vi "GUI_HTT_MultiCamDriveGaiaProfile.vi"() -> ()   [LabVIEW 2020]
uses:
  Shared/GUI_Template/GUI_master/tcp_new_data_event.ctl
  Shared/GUI_Template/GUI_master/tcp new data cluster.ctl
  General GUIs/Device GUIs/GUI_Cameras/Controls/Crosshair type def.ctl
  <userlib>/_OpenG.lib/array/array.llb/Filter 1D Array with Scalar (String)__ogtk.vi
panel:
  out "String 4":string="x1\ny1\nx2\ny2"
  out "String 3":string="x1\ny1\nx2\ny2"
  out "String 2":string="x1\ny1\nx2\ny2"
  out "String":string="x1\ny1\nx2\ny2"
  in  "visibility":bool=TRUE
  out "appended array":string[](array[string]) caption="XH"
  out "appended array 6":string[](array[string]) caption="XH"
  out "appended array 8":string[](array[string]) caption="XH"
  out "appended array 4":string[](array[string]) caption="XH"
  in  "UDP error message":string
  out "tcp data event 2":T1
  out "error IO 2":errorcluster
  in  "Color Box":u32(colorbox)
  in  "TargetSize.Y::3":dbl=163.0 caption="y" min=2.0 max=3000.0 format="%#_6f"
  in  "TargetSize.X::3":dbl=152.0 caption="x" min=2.0 max=3000.0 format="%#_6f"
  in  "TargetSize.Y::2":dbl=74.0 caption="y" min=2.0 max=3000.0 format="%#_6f"
  in  "TargetSize.X::2":dbl=75.0 caption="x" min=2.0 max=3000.0 format="%#_6f"
  in  "active cams":string
  out "CCDs":string[](array[string])
  out "Cameras":T2
  in  "Target.Y::3":dbl=163.0 caption="y" min=0.0 max=2000.0 format="%#_6f"
  in  "Target.X::3":dbl=152.0 caption="x" min=0.0 max=2000.0 format="%#_6f"
  in  "Target.Y::2":dbl=74.0 caption="y" min=0.0 max=2000.0 format="%#_6f"
  in  "Target.X::2":dbl=75.0 caption="x" min=0.0 max=2000.0 format="%#_6f"
  out "error out":errorcluster
  in  "triggerdelay::3":dbl=0.001 caption="triggerdelay" min=0.0 max=10000000.0 format="%_4p"
  in  "triggerdelay::2":dbl=0.001 caption="triggerdelay" min=0.0 max=10000.0 format="%_4p"
  in  "centroidy::5":dbl=0.001 caption="centroid y" min=0.0 max=0.0 format="%_4f"
  in  "centroidx::5":dbl=0.001 caption="centroid x" min=0.0 max=0.0 format="%_4f"
  in  "trigger::3":bool caption="Trigger"
  in  "centroidy::3":dbl=0.001 caption="centroid y" min=0.0 max=0.0 format="%_4f"
  in  "centroidx::3":dbl=0.001 caption="centroid x" min=0.0 max=0.0 format="%_4f"
  in  "exposure::3":dbl=0.001 caption="exposure" min=1e-07 max=5.0 format="%_4p"
  out "image::3":T3(plugin-control) caption="HTT-MagCam-03"
  in  "GUIdevice 3":string="HTT-C24_1_gmode_n"
  in  "trigger::2":bool caption="Trigger"
  in  "centroidy::2":dbl=0.001 caption="centroid y" min=0.0 max=0.0 format="%_4f"
  in  "centroidx::2":dbl=0.001 caption="centroid x" min=0.0 max=0.0 format="%_4f"
  in  "exposure::2":dbl=0.001 caption="exposure" min=0.0001 max=1.0 format="%_4p"
  out "image::2":T3(plugin-control) caption="HTT-MagCam-04"
  in  "GUIdevice 2":string="HTT-C13_4_gmode_s"
  out "tcp data event":T1
  in  "Refresh Button":bool caption="Update Crosshairs"
  in  "Select device":string(combo)="FrogHPD"
  in  "stop":bool
  in  "GUIdevice 1":string="HPD_CCD"
  # "XHair location"
  # "XHair location"
  # "XHair size"
  # "XHair size"
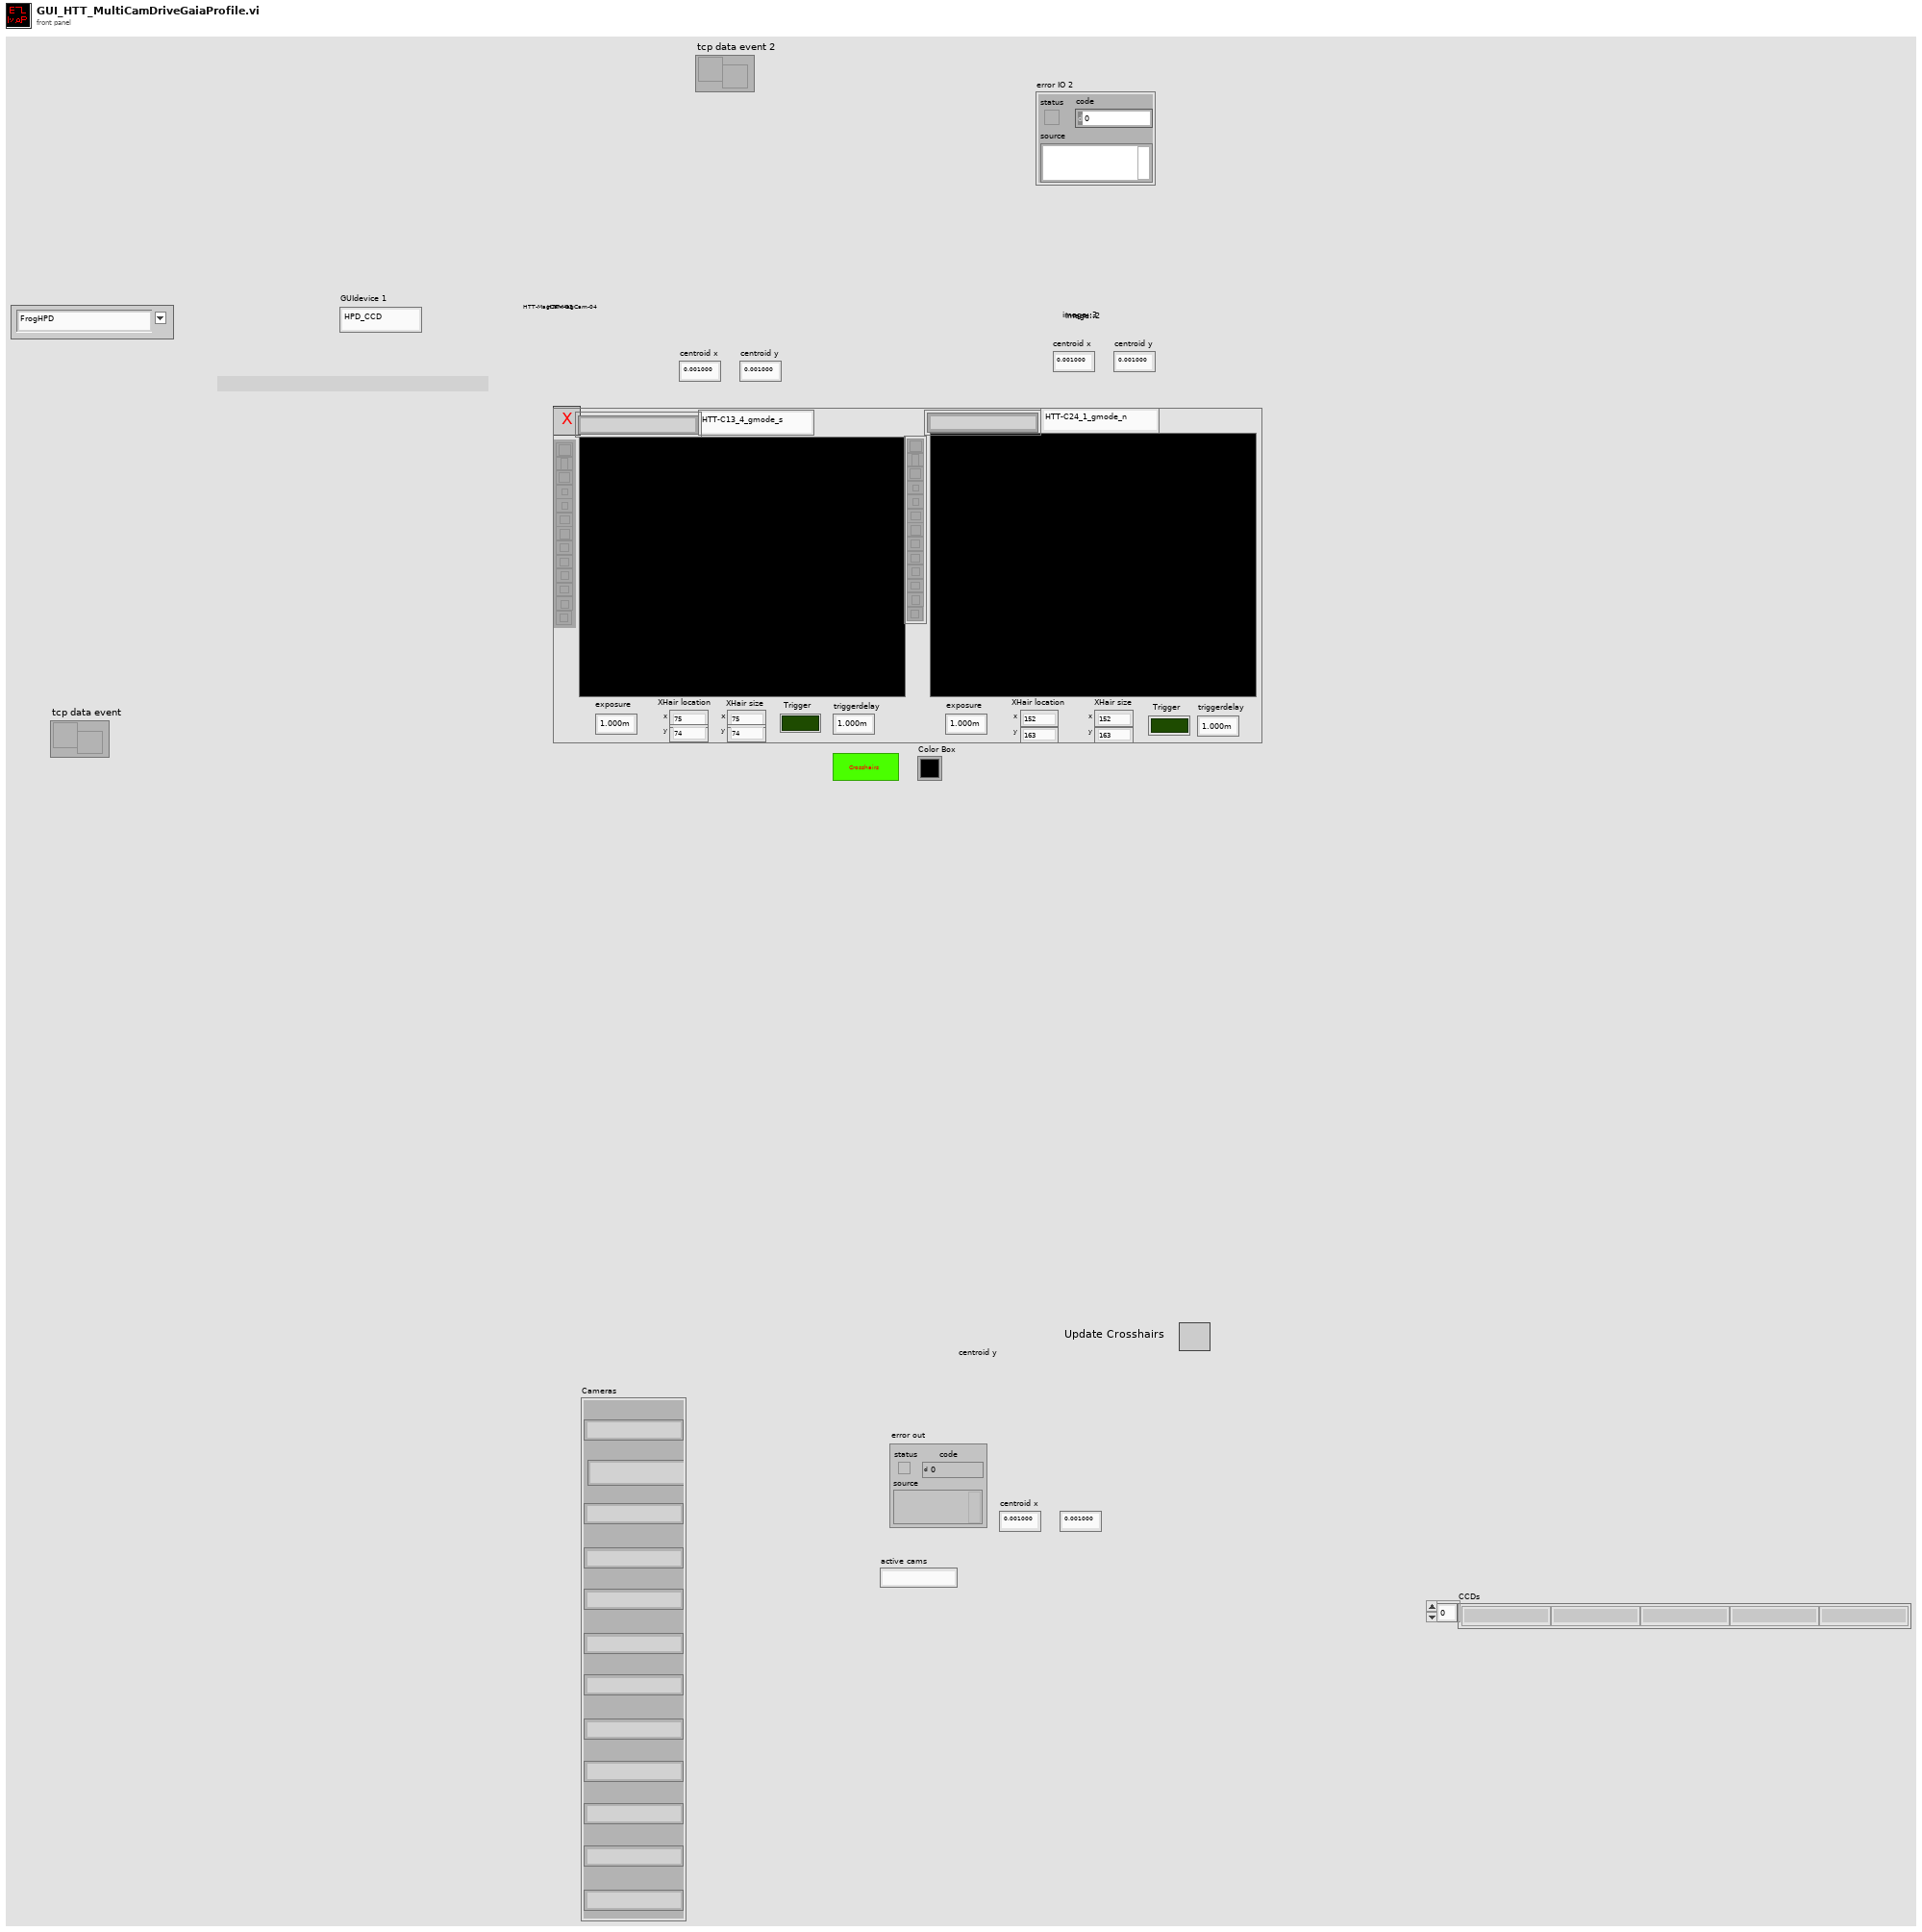
[diagram p1: front panel]
types:
  T1 = typedef "tcp_new_data_event.ctl" = refnum<user-event>
  T2 = cluster{"[0]":string, "[1]":string, "[2]":string, "[3]":string, "[4]":string, "[5]":string, "[6]":string, "[7]":string, "[8]":string, "[8] 2":string, "[8] 3":string, "[8] 4":string}
  T3 = typedef "IMAQ Image.ctl" = refnum<image>
  T4 = typedef "Image Type" = u32
  T5 = cluster{"Target.X::2":refnum<vi>, "Target.Y::2":refnum<vi>}
  T6 = cluster{"Target.X::3":refnum<vi>, "Target.Y::3":refnum<vi>}
  T7 = cluster{"TargetSize.X::2":refnum<vi>, "TargetSize.Y::2":refnum<vi>}
  T8 = cluster{"TargetSize.X::3":refnum<vi>, "TargetSize.Y::3":refnum<vi>}
  T9 = cluster{"Target.X::3":refnum<vi>, "Target.Y::3":refnum<vi>}[]
  T10 = cluster{"TargetSize.X::3":refnum<vi>, "TargetSize.Y::3":refnum<vi>}[]
  T11 = cluster{"[0]":string, "[1]":string, "[2]":string, "[3]":string, "[4]":string, "[5]":string, "[6]":string, "[7]":string, "[8]":string, "[9]":string, "[10]":string, "[11]":string}
  T12 = typedef "Crosshair type def.ctl" = cluster{"Draw":bool, "Target":cluster{"x":dbl, "y":dbl}, "Size":cluster{"x":dbl, "y":dbl}, "Angle":dbl, "Color":u32, "Thickness":u8, "CrosshairLabel":string}
  T13 = cluster{"Left":i32, "Top":i32, "Right":i32, "Bottom":i32}
  T14 = enum32{"invalid app kind", "Development System", "Run Time System", "Student Edition", "Embedded LabVIEW", "Evaluation", "Custom"}
  T15 = typedef "tcp new data cluster.ctl" = cluster{"EventEnum":enum16{"new data", "connection status update"}, "Device name":string}
  T16 = enum32{"Invalid", "Standard", "Closed", "Hidden", "Minimized", "Maximized"}
  T17 = cluster{"Core":cluster{"Current VI Reference":refnum<vi>, "Close Panel on Exit?":bool}, "Your Boolean data":bool, "active cams":string, "SuperGUI":cluster{"STOP queue":refnum<queue>, "SuperGUI ref":refnum<vi>}}
  T18 = cluster{"STOP queue":refnum<queue>, "SuperGUI ref":refnum<vi>}
  T19 = cluster{"Current VI Reference":refnum<vi>, "Close Panel on Exit?":bool}
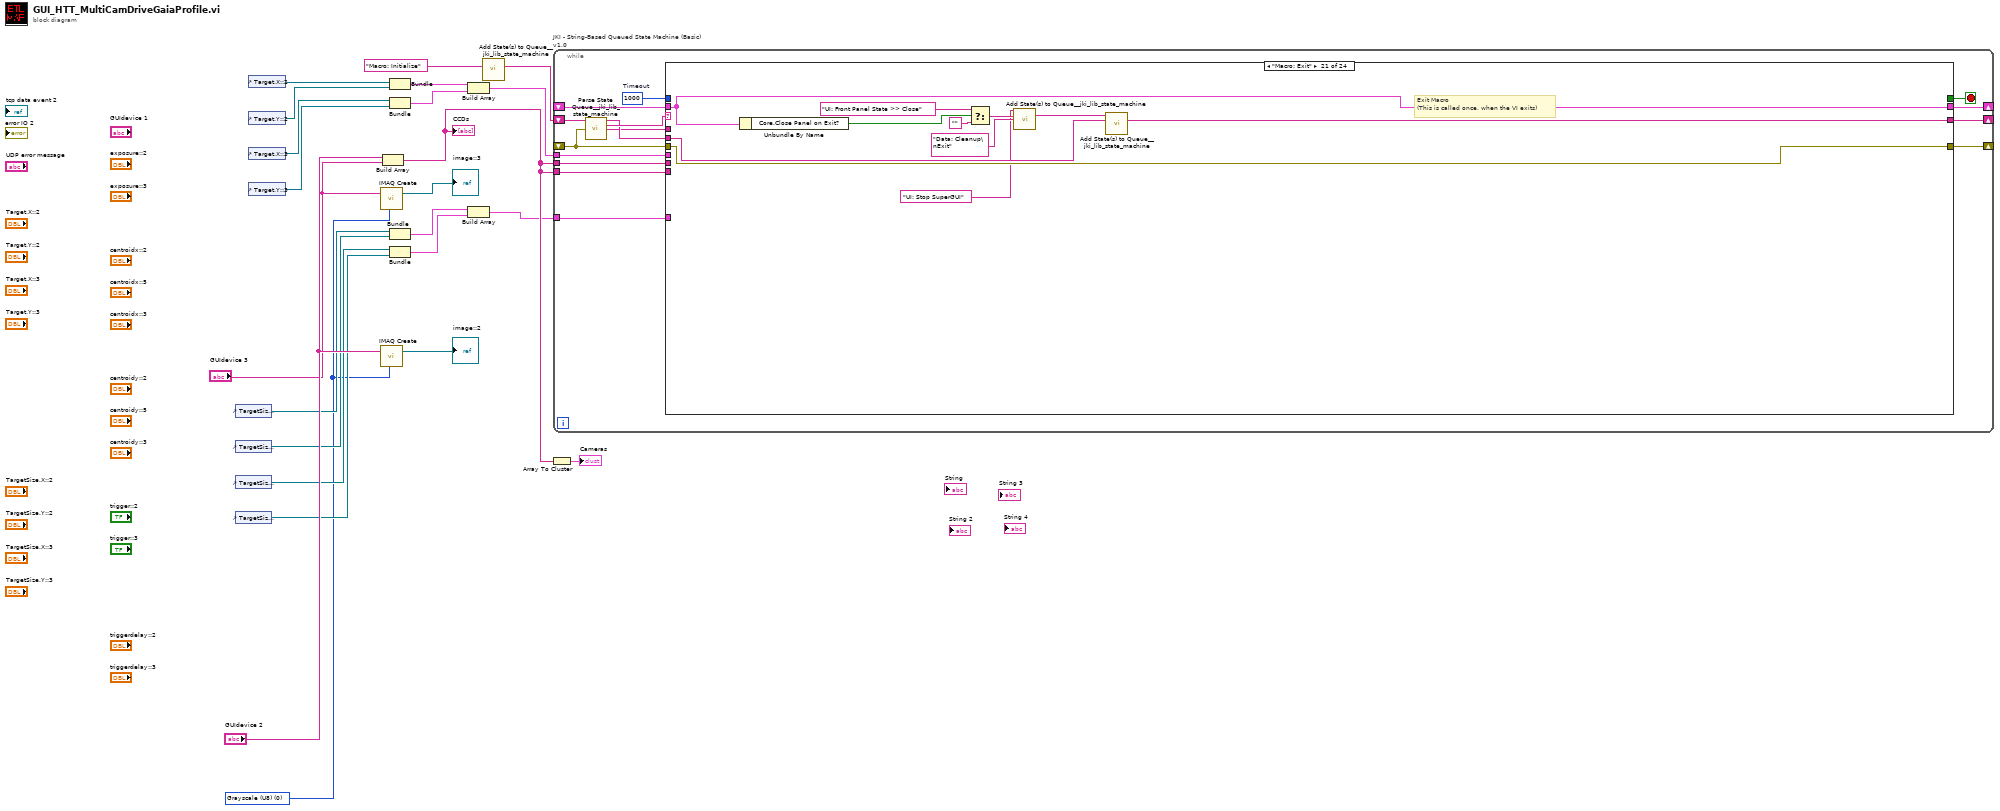
[diagram p0: block diagram]
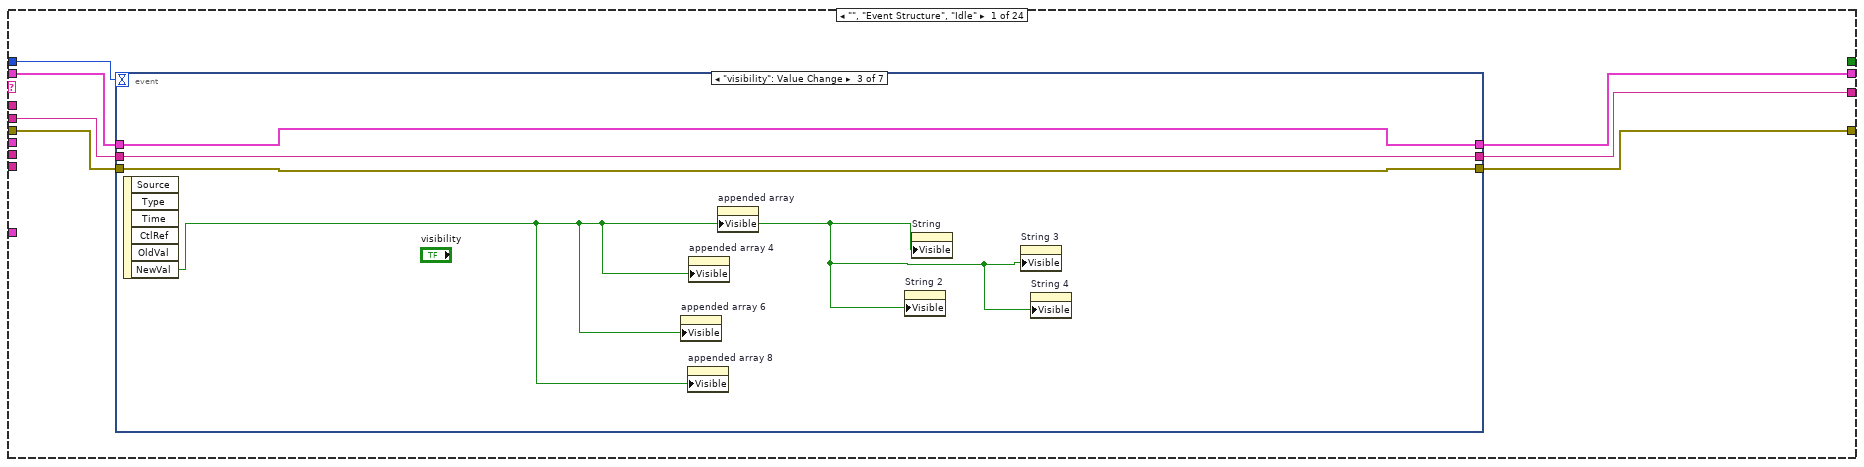
[diagram p2: hidden frame]
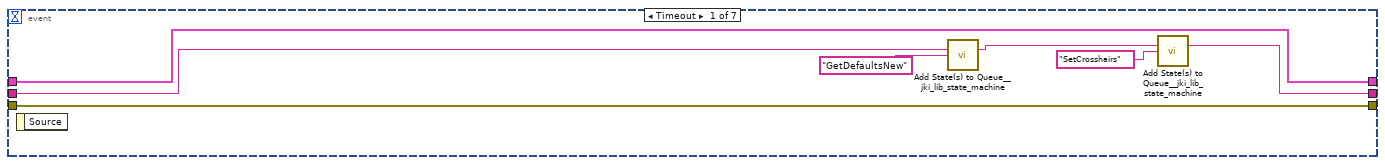
[diagram p3: hidden frame]
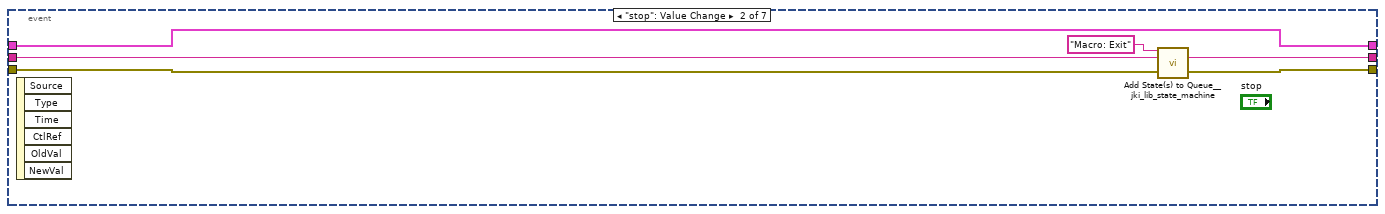
[diagram p4: hidden frame]
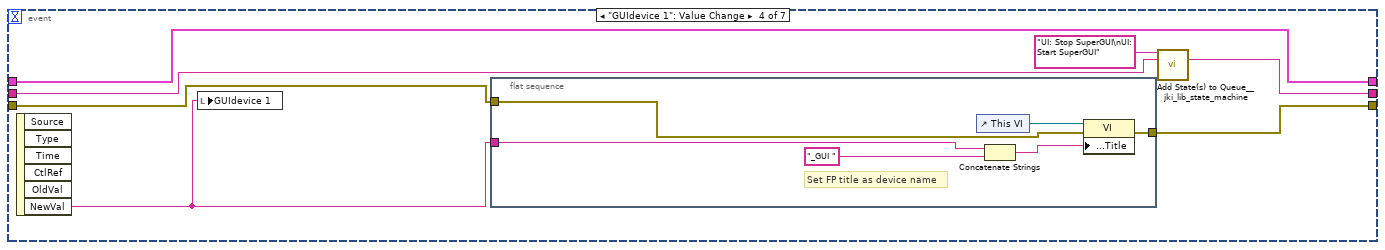
[diagram p5: hidden frame]
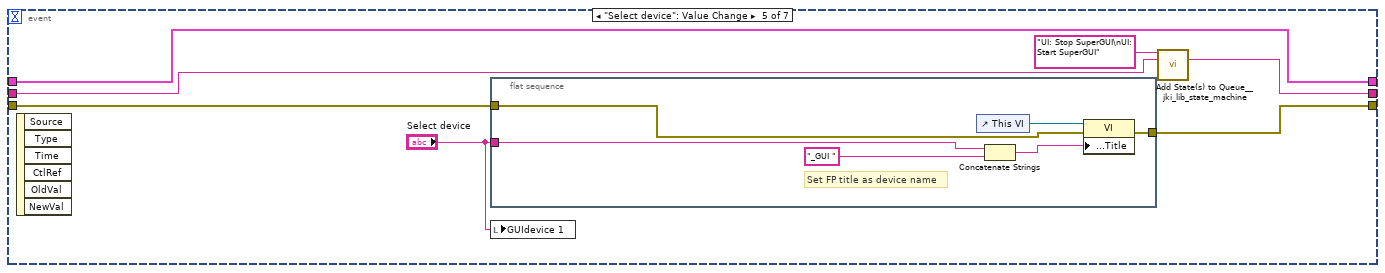
[diagram p6: hidden frame]
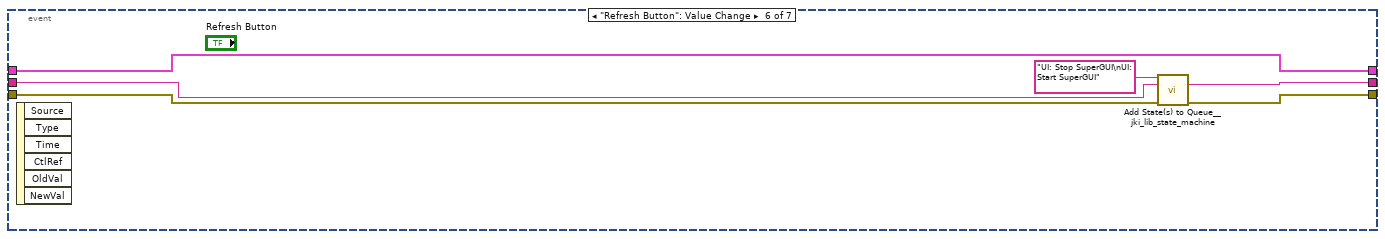
[diagram p7: hidden frame]
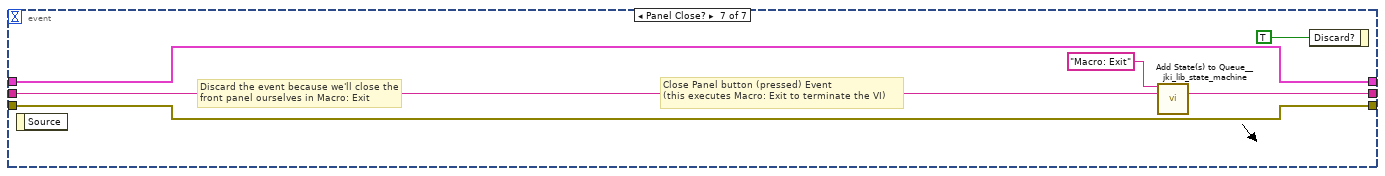
[diagram p8: hidden frame]
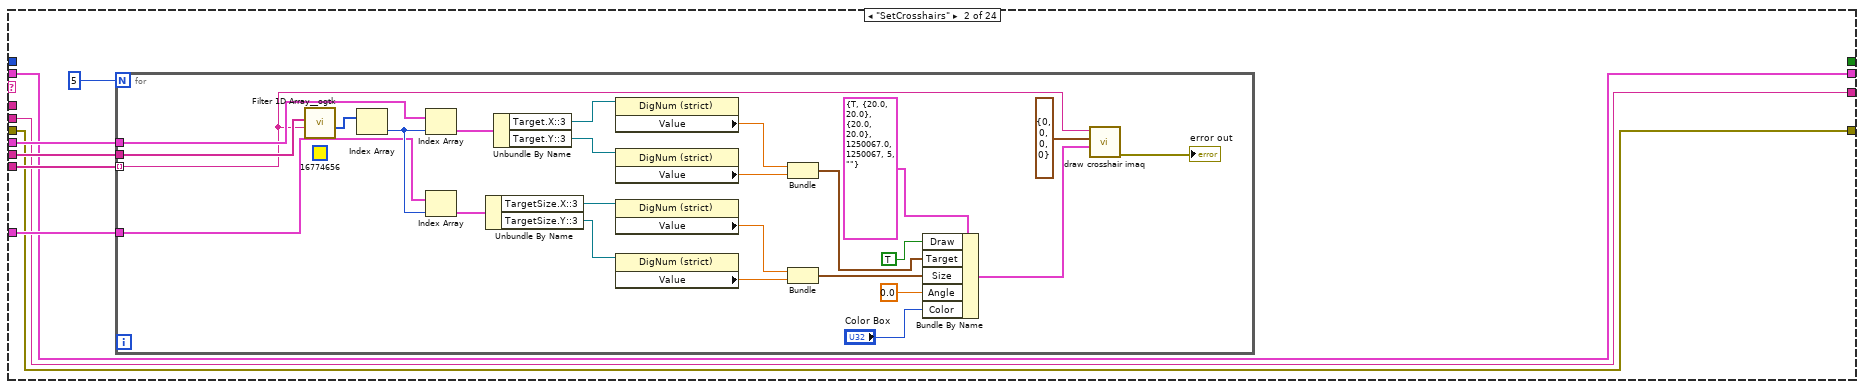
[diagram p9: hidden frame]
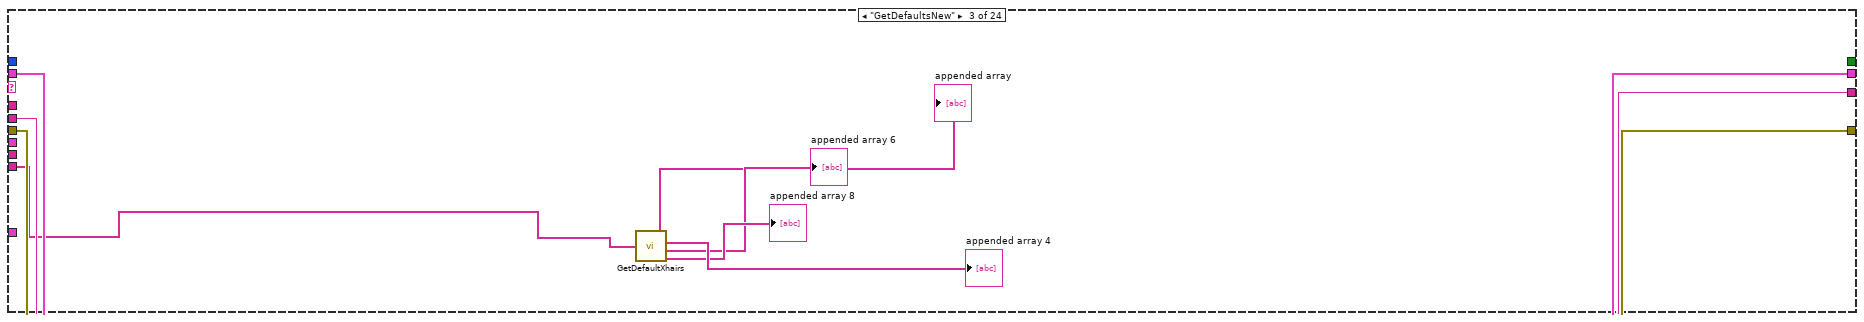
[diagram p10: hidden frame]
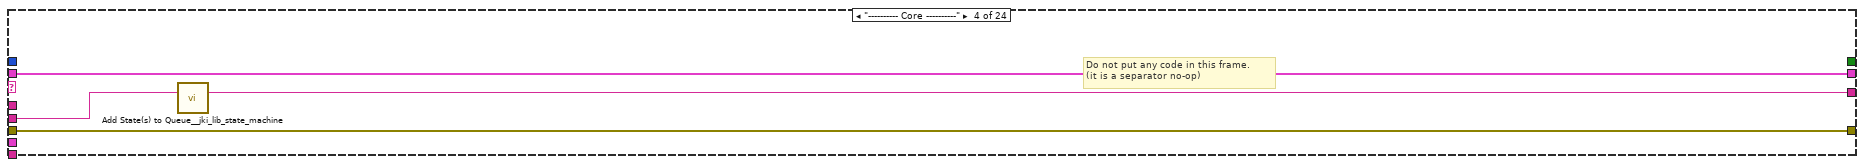
[diagram p11: hidden frame]
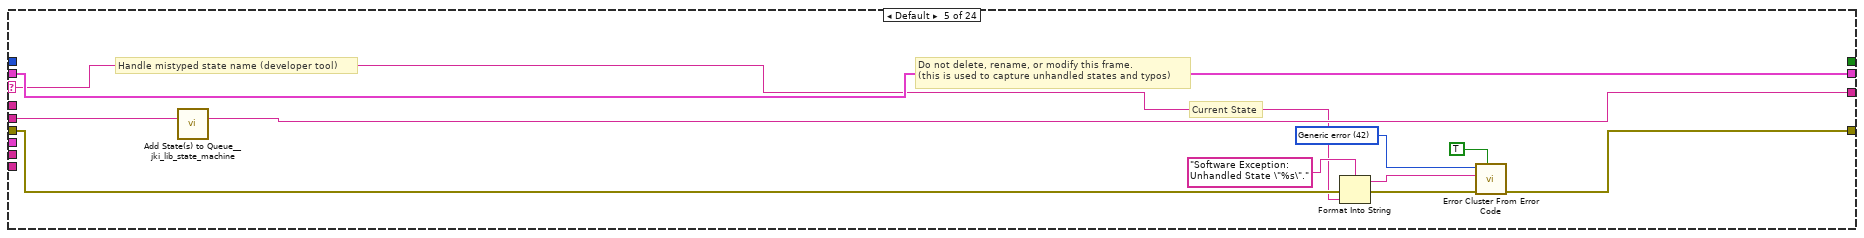
[diagram p12: hidden frame]
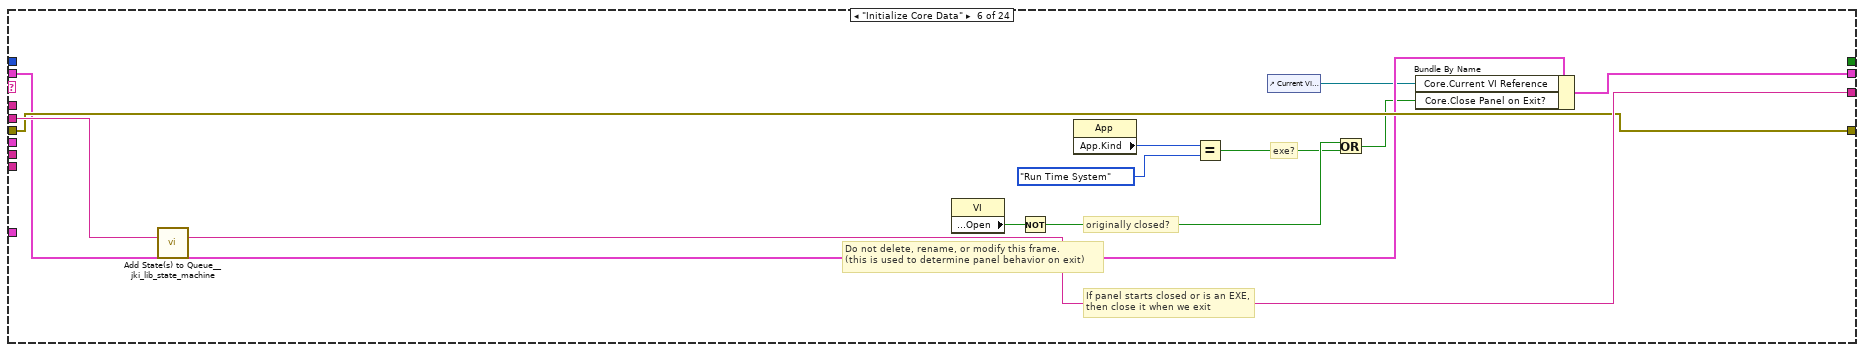
[diagram p13: hidden frame]
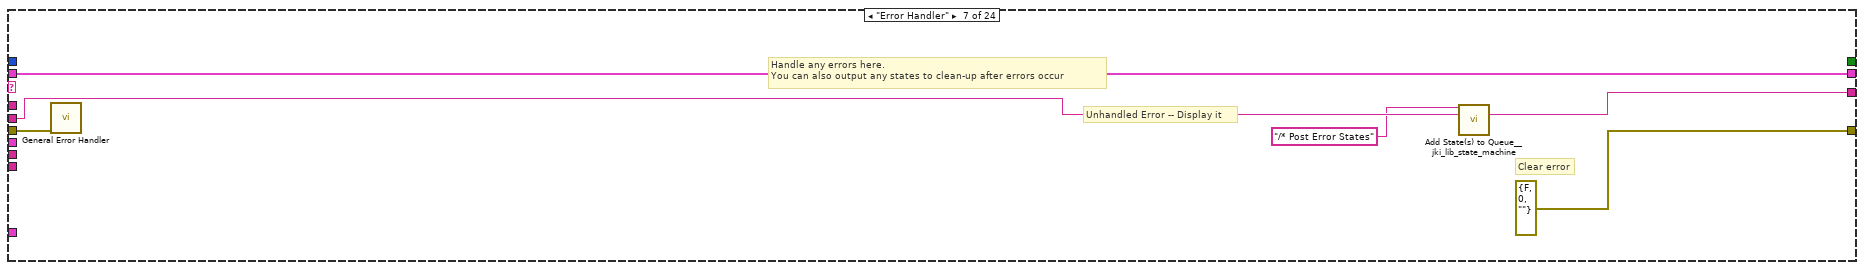
[diagram p14: hidden frame]
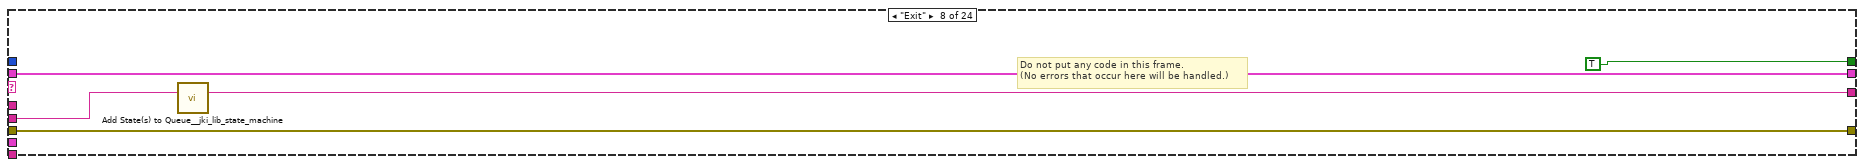
[diagram p15: hidden frame]
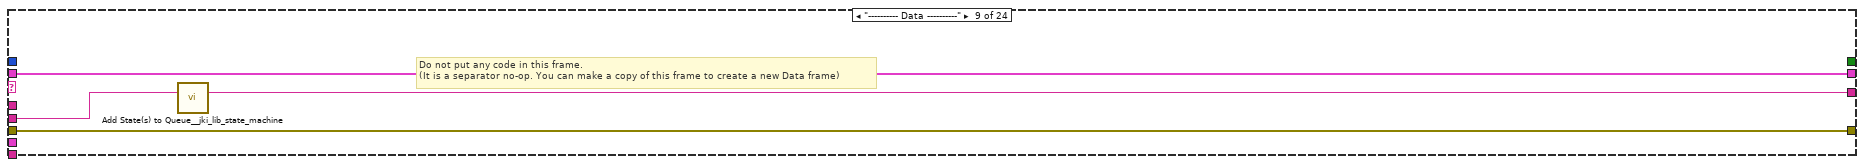
[diagram p16: hidden frame]
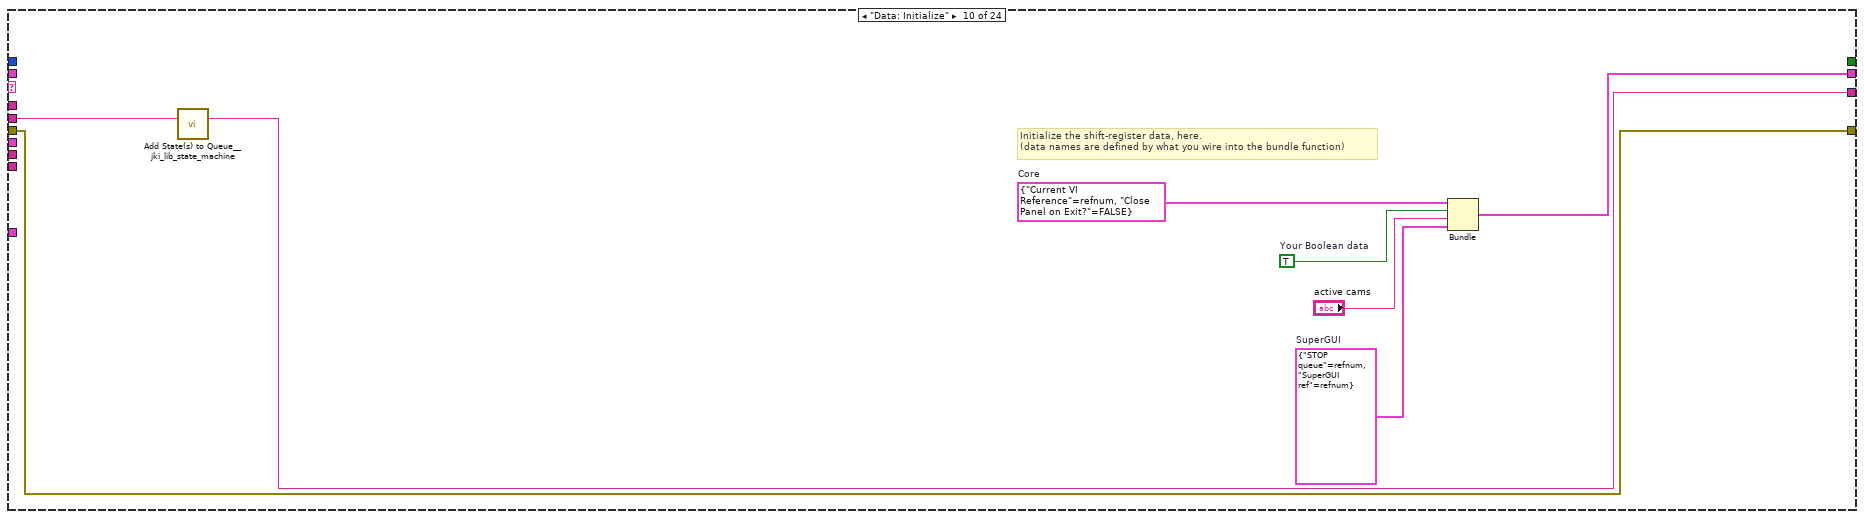
[diagram p17: hidden frame]
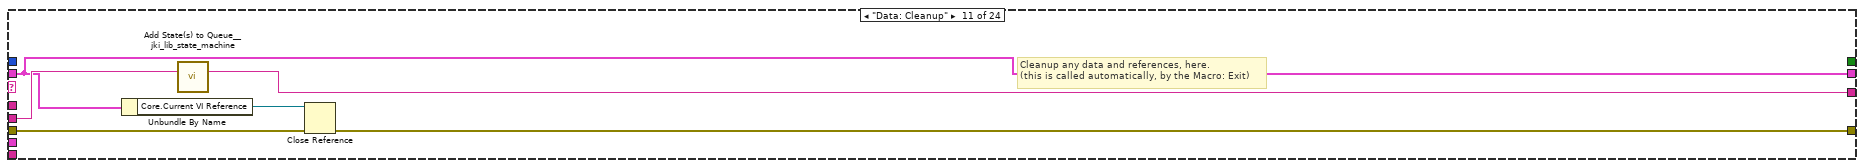
[diagram p18: hidden frame]
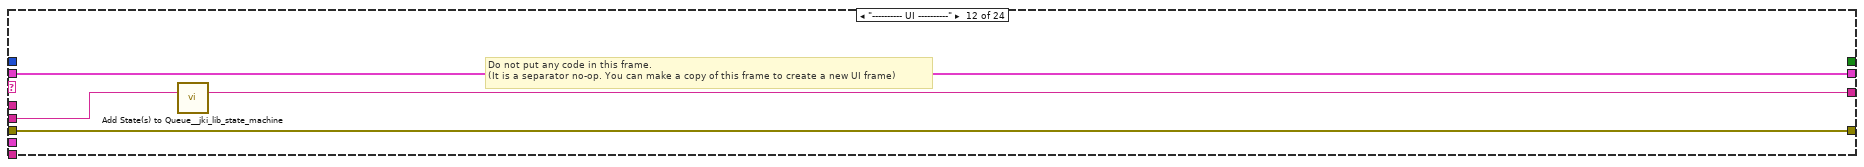
[diagram p19: hidden frame]
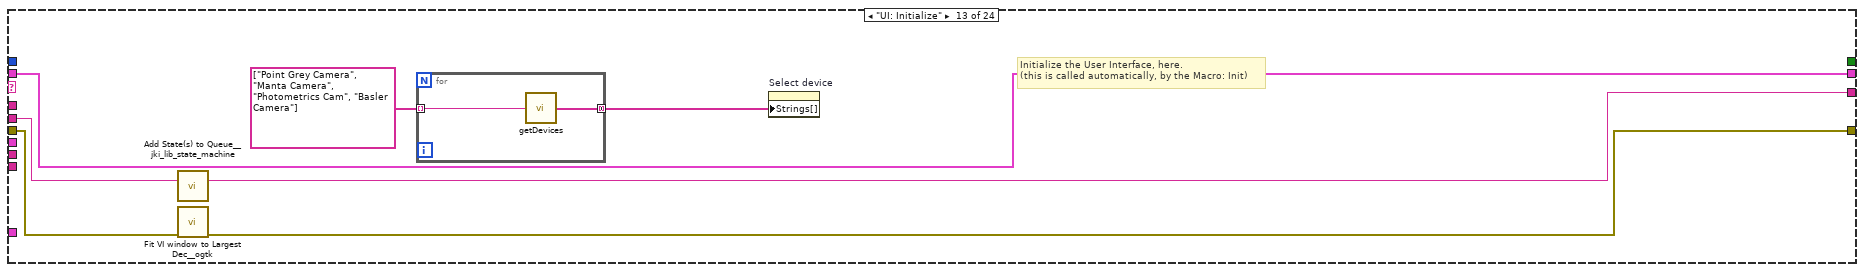
[diagram p20: hidden frame]
diagram:
  w1 = T4 0 items=["Grayscale (U8)", "Grayscale (I16)", "Grayscale (SGL)", "Complex (CSG)", "RGB (U32)", "HSL (U32)", "RGB (U64)", "Grayscale (U16)"] ("Image Type")
  n1 = control-ref of="TargetSize.X::2"() -> (w8:refnum<vi>)
  n2 = control-ref of="TargetSize.Y::2"() -> (w7:refnum<vi>)
  n3 = control-ref of="TargetSize.X::3"() -> (w6:refnum<vi>)
  n4 = control-ref of="TargetSize.Y::3"() -> (w5:refnum<vi>)
  n5 = control-ref of="Target.X::2"() -> (w19:refnum<vi>)
  n6 = control-ref of="Target.Y::2"() -> (w18:refnum<vi>)
  n7 = control-ref of="Target.X::3"() -> (w17:refnum<vi>)
  n8 = control-ref of="Target.Y::3"() -> (w16:refnum<vi>)
  n9 = call "IMAQ Create"("Image Name"="GUIdevice 3", "Image Type"=w1) -> ("New Image"=→"image::3":T3)  [unwired: 3 in, 1 out]
  n10 = call "IMAQ Create"("Image Name"="GUIdevice 2", "Image Type"=w1) -> ("New Image"=→"image::2":T3)  [unwired: 3 in, 1 out]
  n11 = Build Array("GUIdevice 2", "GUIdevice 3") -> (w9:string[])
  "CCDs" <- w9
  n12 = Bundle("Target.X::2"=w19, "Target.Y::2"=w18) -> (w15:T5)  [unwired: 1 in]
  n13 = Bundle("Target.X::3"=w17, "Target.Y::3"=w16) -> (w14:T6)  [unwired: 1 in]
  n14 = Bundle("TargetSize.X::2"=w8, "TargetSize.Y::2"=w7) -> (w4:T7)  [unwired: 1 in]
  n15 = Bundle("TargetSize.X::3"=w6, "TargetSize.Y::3"=w5) -> (w3:T8)  [unwired: 1 in]
  n16 = Build Array(w15, w14) -> (w13:T9)
  n17 = Build Array(w4, w3) -> (w2:T10)
  n18 = call <vilib>:"Add State(s) to Queue__jki_lib_state_machine.vi"("State(s) in (\"\")"="Macro: Initialize") -> ("States Out"=w23:string)  [unwired: 14 in]
  n19 = Array To Cluster(array=w9) -> (cluster=→"Cameras":T11)
  n20 = while "JKI - String-Based Queued State Machine (Basic) v1.0" {
    shift-right: [w31] -> _
    shift-left: _ -> [w28]
    shift-right: [w34] -> _
    shift-left: _ -> [w29]
    shift-right: [w33] -> _
    shift-left: w23 -> [w35]
    tunnel: w13 -> [w25]
    tunnel: w9 -> [w26]
    tunnel: w9 -> [w27]
    tunnel: w2 -> [w24]
    stop <- w32 stop-if-true
    w30 = 1000  # Timeout
    n21 = call <vilib>:"Parse State Queue__jki_lib_state_machine.vi"("State Queue"=w35, "Error In (no error)"=w29) -> ("Remaining States"=w37:string, "Current State"=w38:string, "Arguments"=w36:string)  [unwired: 11 in]
    n22 = case shown="\"Macro: Exit\"" w38 {
      selector: w38 -> [_ _ _ _ w144 _ _ _ _ _ _ _ _ _ _ _ _ _ _ _ _ _ _ _]
      tunnel: w37 -> [w45 w101 w138 w143 w148 w166 w172 w177 w181 w189 w195 w199 w206 w214 w249 w257 w263 w274 w300 w305 w316 w320 w324 w328]
      tunnel: w36 -> [_ _ _ _ _ _ _ _ _ _ _ _ _ _ _ _ w258 w268 _ _ _ _ _ _]
      tunnel: w28 -> [w43 w102 w139 w140 w146 w157 w169 w175 w178 _ w190 w196 w204 w212 w240 w252 w261 w270 w297 w302 w313 w317 w321 w325]
      tunnel: [w42 w100 w137 w141 w150 w163 errorcluster {"status"=FALSE, "code"=0, "source"=""} ("error out") w174 w179 w186 w191 w197 w202 w209 w233 w250 w259 w271 w298 w303 w314 w318 w322 w326] -> w34
      tunnel: w29 -> [w41 w100 w137 w141 w149 w163 w168 w174 w179 w186 w192 w197 w203 w210 w234 w251 w260 w272 w298 w303 w314 w318 w322 w326]
      tunnel: [w44 w101 w138 w142 w147 w165 w171 w176 w180 w188 w194 w198 w205 w213 w248 w256 w262 w273 w299 w304 w315 w319 w323 w327] -> w33
      tunnel: [_ _ _ _ _ _ _ TRUE _ _ _ _ _ _ _ _ _ _ _ _ _ _ _ _] -> w32
      tunnel: [w40 w102 w139 w140 w146 w164 w169 w175 w178 w187 w190 w196 w204 w212 w239 w252 w261 w270 w297 w302 w313 w317 w321 w325] -> w31
      tunnel: w30 -> [w39 _ _ _ _ _ _ _ _ _ _ _ _ _ _ _ _ _ _ _ _ _ _ _]
      tunnel: w27 -> [_ w104 w136 _ _ _ _ _ _ _ _ _ _ _ _ _ _ _ _ _ _ _ _ _]
      tunnel: w26 -> [_ w105 _ _ _ _ _ _ _ _ _ _ _ _ _ _ _ _ _ _ _ _ _ _]
      tunnel: w25 -> [_ w106 _ _ _ _ _ _ _ _ _ _ _ _ _ _ _ _ _ _ _ _ _ _]
      tunnel: w24 -> [_ w103 _ _ _ _ _ _ _ _ _ _ _ _ _ _ _ _ _ _ _ _ _ _]
      frame "", "Event Structure", "Idle" {
        n23 = event shown="[2] \"visibility\": Value Change" {
          selector: _ -> [_ _ _ _ _ _ _]
          dyn-events: _ -> [_ _ _ _ _ _ _]
          timeout: w39 -> [_ _ _ _ _ _ _]
          tunnel: w45 -> [w48 w55 w59 w65 w77 w90 w98]
          tunnel: [w52 w54 w59 w64 w76 w89 w97] -> w44
          tunnel: w43 -> [w50 w57 w61 w68 w81 w92 w95]
          tunnel: [w51 w56 w60 w66 w79 w91 w96] -> w42
          tunnel: w41 -> [w51 w56 w60 w67 w80 w91 w96]
          tunnel: [w50 w57 w61 w68 w81 w92 w95] -> w40
          event Timeout {
            n24 = event-data() -> ()  [unwired: 1 in, 1 out]
            n25 = call <vilib>:"Add State(s) to Queue__jki_lib_state_machine.vi"("State(s) in (\"\")"=w48, "State(s) at Back (\"\")"="GetDefaultsNew") -> ("States Out"=w46:string)  [unwired: 13 in]
            n26 = call <vilib>:"Add State(s) to Queue__jki_lib_state_machine.vi"("State(s) in (\"\")"=w46, "State(s) at Back (\"\")"="SetCrosshairs") -> ("States Out"=w52:string)  [unwired: 13 in]
          }
          event "stop": Value Change {
            n27 = event-data() -> ()  [unwired: 1 in, 6 out]
            n28 = call <vilib>:"Add State(s) to Queue__jki_lib_state_machine.vi"("State(s) in Front (\"\")"="Macro: Exit", "State(s) in (\"\")"=w55) -> ("States Out"=w54:string)  [unwired: 13 in]
          }
          event "visibility": Value Change {
            n29 = event-data() -> ("NewVal"=w58:bool)  [unwired: 1 in, 5 out]
            n30 = property on="appended array 6" class="Arr (strict)"("Visible"=w58) -> ()  [unwired: 2 in, 2 out]
            n31 = property on="appended array 8" class="Arr (strict)"("Visible"=w58) -> ()  [unwired: 2 in, 2 out]
            n32 = property on="appended array 4" class="Arr (strict)"("Visible"=w58) -> ()  [unwired: 2 in, 2 out]
            n33 = property on="appended array" class="Arr (strict)"("Visible"=w58) -> ()  [unwired: 2 in, 2 out]
            n34 = property on="String 2" class="Str"("Visible"=w58) -> ()  [unwired: 2 in, 2 out]
            n35 = property on="String" class="Str"("Visible"=w58) -> ()  [unwired: 2 in, 2 out]
            n36 = property on="String 3" class="Str"("Visible"=w58) -> ()  [unwired: 2 in, 2 out]
            n37 = property on="String 4" class="Str"("Visible"=w58) -> ()  [unwired: 2 in, 2 out]
          }
          event "GUIdevice 1": Value Change {
            n38 = event-data() -> ("NewVal"=w62:string)  [unwired: 1 in, 5 out]
            n39 = local write "GUIdevice 1"(w62) -> ()
            n40 = flat-sequence {
              tunnel: [w71] -> w66
              tunnel: w67 -> [w70]
              tunnel: w62 -> [w69]
              frame #0 {
                # "Set FP title as device name"
                n41 = control-ref of="This VI"() -> (w74:refnum<vi>)
                n42 = Concatenate Strings(w69, "_GUI ") -> (w73:string)
                n43 = property class="VI"(reference=w74, error in=w70, "Front Panel.Title"=w73) -> (error out=w71:errorcluster)  [unwired: 1 out]
              }
            }
            n44 = call <vilib>:"Add State(s) to Queue__jki_lib_state_machine.vi"("State(s) in Front (\"\")"="UI: Stop SuperGUI\nUI: Start SuperGUI", "State(s) in (\"\")"=w65) -> ("States Out"=w64:string)  [unwired: 13 in]
          }
          event "Select device": Value Change {
            n45 = event-data() -> ()  [unwired: 1 in, 6 out]
            n46 = flat-sequence {
              tunnel: [w84] -> w79
              tunnel: w80 -> [w83]
              tunnel: "Select device" -> [w82]
              frame #0 {
                # "Set FP title as device name"
                n47 = control-ref of="This VI"() -> (w87:refnum<vi>)
                n48 = Concatenate Strings(w82, "_GUI ") -> (w86:string)
                n49 = property class="VI"(reference=w87, error in=w83, "Front Panel.Title"=w86) -> (error out=w84:errorcluster)  [unwired: 1 out]
              }
            }
            n50 = local write "GUIdevice 1"("Select device") -> ()
            n51 = call <vilib>:"Add State(s) to Queue__jki_lib_state_machine.vi"("State(s) in Front (\"\")"="UI: Stop SuperGUI\nUI: Start SuperGUI", "State(s) in (\"\")"=w77) -> ("States Out"=w76:string)  [unwired: 13 in]
          }
          event "Refresh Button": Value Change {
            n52 = event-data() -> ()  [unwired: 1 in, 6 out]
            n53 = call <vilib>:"Add State(s) to Queue__jki_lib_state_machine.vi"("State(s) in Front (\"\")"="UI: Stop SuperGUI\nUI: Start SuperGUI", "State(s) in (\"\")"=w90) -> ("States Out"=w89:string)  [unwired: 13 in]
          }
          event Panel Close? {
            # "Discard the event because we'll close the front panel ourselves in Macro: Exit"
            # "Close Panel button (pressed) Event\n(this executes Macro: Exit to terminate the VI)"
            n54 = event-data() -> ()  [unwired: 1 in, 1 out]
            n55 = call <vilib>:"Add State(s) to Queue__jki_lib_state_machine.vi"("State(s) in Front (\"\")"="Macro: Exit", "State(s) in (\"\")"=w98) -> ("States Out"=w97:string)  [unwired: 13 in]
            n56 = event-data("Discard?"=TRUE) -> ()  [unwired: 1 in, 1 out]
          }
        }
      }
      frame "SetCrosshairs" {
        n57 = for {
          N: 5 -> [_]
          tunnel: w105 -> [w110]
          tunnel: w106 -> [w109]
          tunnel: w103 -> [w108]
          tunnel: w104 -> [w107] mode=indexing
          (unwired) u32 16774656 ("Color")
          n58 = call-poly <userlib>:"Filter 1D Array__ogtk.vi"("items to filter"=w107, "array"=w110) -> ("filtered item indices"=w114:i32[])  [unwired: 4 in, 1 out]
          n59 = Index Array(array=w114) -> (element=w117:i32)  [unwired: 1 in]
          n60 = Index Array(array=w109, index=w117) -> (element=w115:T6)
          n61 = Index Array(array=w108, index=w117) -> (element=w118:T8)
          n62 = Unbundle By Name(w118) -> ("TargetSize.X::3"=w119:refnum<vi>, "TargetSize.Y::3"=w120:refnum<vi>)
          n63 = Unbundle By Name(w115) -> ("Target.X::3"=w112:refnum<vi>, "Target.Y::3"=w113:refnum<vi>)
          n64 = property class="DigNum (strict)"(reference=w112) -> ("Value"=w126:dbl)  [unwired: 1 in, 2 out]
          n65 = property class="DigNum (strict)"(reference=w113) -> ("Value"=w127:dbl)  [unwired: 1 in, 2 out]
          n66 = property class="DigNum (strict)"(reference=w119) -> ("Value"=w121:dbl)  [unwired: 1 in, 2 out]
          n67 = property class="DigNum (strict)"(reference=w120) -> ("Value"=w122:dbl)  [unwired: 1 in, 2 out]
          n68 = Bundle("Value"=w126, "Value"=w127) -> (w128:cluster{"Value":dbl, "Value":dbl})  [unwired: 1 in]
          n69 = Bundle("Value"=w121, "Value"=w122) -> (w129:cluster{"Value":dbl, "Value":dbl})  [unwired: 1 in]
          n70 = Bundle By Name(cluster=T12 {"Draw"=TRUE, "Target"={"x"=20.0, "y"=20.0}, "Size"={"x"=20.0, "y"=20.0}, "Angle"=1250067.0, "Color"=1250067, "Thickness"=5, "CrosshairLabel"=""} ("Crosshair"), "Draw"=TRUE, "Target"=w128, "Size"=w129, "Angle"=0.0, "Color"="Color Box") -> (w124:T12)
          n71 = call "draw crosshair imaq.vi"("Crosshair"=w124, "Bounding Rectangle"=T13 {"Left"=0, "Top"=0, "Right"=0, "Bottom"=0}, "image in"=w107) -> ("error out"=→"error out":errorcluster)  [unwired: 7 in, 1 out]
        }
      }
      frame "GetDefaultsNew" {
        n72 = call "GetDefaultXhairs.vi"("appended array 2"=w136) -> ("appended array"=→"appended array":string[], "appended array 4"=→"appended array 4":string[], "appended array 6"=→"appended array 6":string[], "appended array 8"=→"appended array 8":string[])
      }
      frame "---------- Core ----------" {
        # "Do not put any code in this frame.\n(it is a separator no-op)"
        n73 = call <vilib>:"Add State(s) to Queue__jki_lib_state_machine.vi"("State(s) in (\"\")"=w143) -> ("States Out"=w142:string)  [unwired: 14 in]
      }
      frame Default {
        w153 = 42 items=["No error", "Argument error", "Memory is full", "Out of zone", "End of file", "File already open", "Generic file I/O error", "File not found", "File permission error", "Disk is full", "Duplicate path", "Too many files open", "System feature not enabled", "Resource file not found", "Cannot add resource", "Resource not found", "Image not found", "Image memory error", "Pen does not exist", "Config type invalid", "Config token not found", "Config parse error", "Config memory error", "Bad external code format", "Bad external code offset", "External code not present", "Null window", "Destroy window error", "Null menu", "Print aborted", "Bad print record", "Print driver error", "Windows error during printing", "Memory error during printing", "Print dialog error", "Generic print error", "Invalid device refnum", "Device not found", "Device parameter error", "Device unit error", "Cannot open device", "Device call aborted", "Generic error", "Cancelled by user", "Object ID too low", "Object ID too high", "Object not in heap", "Unknown heap", "Unknown object (invalid DefProc)", "Unknown object (DefProc not in table)", "Message out of range", "Invalid (null) method", "Unknown message", "Manager call not supported", "Bad address", "Network operation in progress", "Network operation timed out", "Connection is busy", "Network attribute not supported", "Network error", "Address in use", "System out of memory", "Connection aborted", "Connection refused", "Not connected", "Already connected", "Connection closed", "Initialization error (interapplication manager)", "Bad occurrence", "Wait on unbound occurrence handler", "Occurrence queue overflow", "Datalog type conflict", "Unused", "Unrecognized type (interapplication manager)", "Memory corrupt", "Failed to make temporary DLL", "Old CIN version", "Drag socket not found", "Failed to load drop-object", "Failed to register OLE object", "Failed to release OLE object", "Format specifier type mismatch", "Unknown format specifier", "Too few format specifiers", "Too many format specifiers", "Scan failed", "Newer CIN version", "Error converting to variant", "Runtime menu error", "Password tampered", "Variant attribute not found", "Incompatible variant data type", "Event data is not available", "Event Store is not present", "Occurrence is not found", "Event Queue is not created", "Event info is not available", "Refnum passed is NULL", "Error retrieving Class GUID", "Error retrieving CoClass GUID", "Error retrieving TypeLib GUID.", "Bad built application magic bytes.", "Specific driver is different from the specific driver associated with the Logical Name.", "There is no session opened to the class driver.", "Max Error", "MAX - Error with config objects", "MAX - Error loading configuration", "MAX - Group not supported"]
        # "Current State"
        # "Do not delete, rename, or modify this frame.\n(this is used to capture unhandled states and typos)"
        # "Handle mistyped state name (developer tool)"
        n74 = call <vilib>:"Add State(s) to Queue__jki_lib_state_machine.vi"("State(s) in (\"\")"=w148) -> ("States Out"=w147:string)  [unwired: 14 in]
        n75 = Format Into String(format string="Software Exception: Unhandled State \"%s\"." ("message"), error in=w149, w144) -> (resulting string=w152:string, error out=w151:errorcluster)  [unwired: 1 in]
        n76 = call <vilib>:"Error Cluster From Error Code.vi"("show call chain? (False)"=TRUE, "error in (no error)"=w151, "error message (\"\")"=w152, "error code (0)"=w153) -> ("error out"=w150:errorcluster)  [unwired: 5 in]
      }
      frame "Initialize Core Data" {
        # "Do not delete, rename, or modify this frame.\n(this is used to determine panel behavior on exit)"
        # "originally closed?"
        # "exe?"
        # "If panel starts closed or is an EXE, then close it when we exit"
        n77 = call <vilib>:"Add State(s) to Queue__jki_lib_state_machine.vi"("State(s) in (\"\")"=w166) -> ("States Out"=w165:string)  [unwired: 14 in]
        n78 = property class="VI"() -> ("Front Panel.Open"=w162:bool)  [unwired: 2 in, 2 out]
        n79 = Not(x=w162) -> (.not. x?=w159:bool)
        n80 = property class="App"() -> ("App.Kind"=w161:T14)  [unwired: 2 in, 2 out]
        n81 = Equal?(x=w161, y=T14."Run Time System" ("Application:Kind")) -> (x = y?=w158:bool)
        n82 = control-ref of="Current VI Reference"() -> (w155:refnum<vi>)
        n83 = Or(x=w159, y=w158) -> (x .or. y?=w156:bool)
        n84 = Bundle By Name(cluster=w157, "Core.Current VI Reference"=w155, "Core.Close Panel on Exit?"=w156) -> (w164:T17)
      }
      frame "Error Handler" {
        # "Unhandled Error -- Display it"
        # "Handle any errors here.\nYou can also output any states to clean-up after errors occur"
        # "Clear error"
        n85 = call <vilib>:"General Error Handler.vi"("error in (no error)"=w168) -> ()  [unwired: 10 in, 5 out]
        n86 = call <vilib>:"Add State(s) to Queue__jki_lib_state_machine.vi"("State(s) in Front (\"\")"="/* Post Error States", "State(s) in (\"\")"=w172) -> ("States Out"=w171:string)  [unwired: 13 in]
      }
      frame "Exit" {
        # "Do not put any code in this frame.\n(No errors that occur here will be handled.)"
        n87 = call <vilib>:"Add State(s) to Queue__jki_lib_state_machine.vi"("State(s) in (\"\")"=w177) -> ("States Out"=w176:string)  [unwired: 14 in]
      }
      frame "---------- Data ----------" {
        # "Do not put any code in this frame.\n(It is a separator no-op. You can make a copy of this frame to create a new Data frame)"
        n88 = call <vilib>:"Add State(s) to Queue__jki_lib_state_machine.vi"("State(s) in (\"\")"=w181) -> ("States Out"=w180:string)  [unwired: 14 in]
      }
      frame "Data: Initialize" {
        w182 = T18 {"STOP queue"=refnum, "SuperGUI ref"=refnum}  # SuperGUI
        w183 = T19 {"Current VI Reference"=refnum, "Close Panel on Exit?"=FALSE}  # Core
        w185 = TRUE  # Your Boolean data
        # "Initialize the shift-register data, here.\n(data names are defined by what you wire into the bundle function)"
        n89 = call <vilib>:"Add State(s) to Queue__jki_lib_state_machine.vi"("State(s) in (\"\")"=w189) -> ("States Out"=w188:string)  [unwired: 14 in]
        n90 = Bundle("Core"=w183, "Your Boolean data"=w185, "active cams"="active cams", "SuperGUI"=w182) -> (w187:T17)  [unwired: 1 in]
      }
      frame "Data: Cleanup" {
        # "Cleanup any data and references, here.\n(this is called automatically, by the Macro: Exit)"
        n91 = Unbundle By Name(w190) -> ("Core.Current VI Reference"=w193:refnum<vi>)
        n92 = call <vilib>:"Add State(s) to Queue__jki_lib_state_machine.vi"("State(s) in (\"\")"=w195) -> ("States Out"=w194:string)  [unwired: 14 in]
        n93 = Close Reference(reference=w193, error in (no error)=w192) -> (error out=w191:errorcluster)
      }
      frame "---------- UI ----------" {
        # "Do not put any code in this frame.\n(It is a separator no-op. You can make a copy of this frame to create a new UI frame)"
        n94 = call <vilib>:"Add State(s) to Queue__jki_lib_state_machine.vi"("State(s) in (\"\")"=w199) -> ("States Out"=w198:string)  [unwired: 14 in]
      }
      frame "UI: Initialize" {
        # "Initialize the User Interface, here.\n(this is called automatically, by the Macro: Init)"
        n95 = call <vilib>:"Add State(s) to Queue__jki_lib_state_machine.vi"("State(s) in (\"\")"=w206) -> ("States Out"=w205:string)  [unwired: 14 in]
        n96 = call <userlib>:"Fit VI window to Largest Dec__ogtk.vi"("error in (no error)"=w203) -> ("error out"=w202:errorcluster)  [unwired: 5 in, 1 out]
        n97 = for {
          tunnel: string[] ["Point Grey Camera", "Manta Camera", "Photometrics Cam", "Basler Camera"] -> [w208] mode=indexing
          tunnel: [w207] -> w200 mode=concatenating
          n98 = call "getDevices.vi"("Device Class"=w208) -> ("All Devices"=w207:string[])
        }
        n99 = property on="Select device" class="CmbBox"("Strings[]"=w200) -> ()  [unwired: 2 in, 2 out]
      }
      frame "UI: Get Device Name" {
        # "Initialize the User Interface, here.\n(this is called automatically, by the Macro: Init)"
        n100 = call <vilib>:"Add State(s) to Queue__jki_lib_state_machine.vi"("State(s) in (\"\")"=w214) -> ("States Out"=w213:string)  [unwired: 14 in]
        n101 = First Call?() -> (First Call?: T/F=w211:bool)
        n102 = case shown="True" w211 {
          tunnel: w210 -> [w215 w217]
          tunnel: [w215 w216] -> w209
          frame False {
          }
          frame True {
            n103 = disable-structure "Get Device name from control for vi mode\nand command line arg for exe" shown="RUN_TIME_ENGINE==True" {
              disable-tunnel: w217 -> [w218 w220]
              disable-tunnel: [w218 w219] -> w216
              frame condition #0 (active) {
              }
              frame condition #1 {
                n104 = control-ref of="This Application"() -> (w228:refnum<vi>)
                n105 = property class="App"(reference=w228) -> ("App.Args"=w227:string[])  [unwired: 1 in, 2 out]
                n106 = Index Array(array=w227, index #1=1 ("index")) -> (element #1=w221:string)  [unwired: 2 in, 2 out]
                n107 = Empty String/Path?(string/path=w221) -> (empty?=w225:bool)
                n108 = Concatenate Strings(w221, "_GUI ") -> (w223:string)
                n109 = case shown="False" w225 {
                  tunnel: w221 -> [w229 _]
                  frame False {
                    n110 = local write "GUIdevice 1"(w229) -> ()
                  }
                  frame True {
                  }
                }
                n111 = control-ref of="This VI"() -> (w224:refnum<vi>)
                n112 = property class="VI"(reference=w224, error in=w220, "Front Panel.Title"=w223) -> (error out=w219:errorcluster)  [unwired: 1 out]
              }
            }
          }
        }
      }
      frame "UI: Start SuperGUI" {
        # "create stop queue for supergui and its clones"
        # "x100 abort will be dependent on caller VI\nx80 abort will be independent of caller vi, this will abort vi when labview is closed."
        # "Start SuperGUI asynchronous way"
        n113 = vi-ref "GUI_Master_subvi_reentrant_queues.vi"() -> (w232:refnum<vi>)
        n114 = property class="VI"(reference=w232) -> ("Path"=w231:path)  [unwired: 1 in, 2 out]
        n115 = control-ref of="This Application"() -> (w238:refnum<vi>)
        n116 = Open VI Reference(type specifier VI Refnum (for type only)=refnum<vi> refnum, vi path=w231, options=256) -> (vi reference=w247:refnum<vi>, error out=w246:errorcluster)  [unwired: 3 in]
        n117 = Create User Event(user event datatype=T15 {"EventEnum"=enum."new data", "Device name"="Device name"} ("New Event"), error in=w234) -> (user event=w235:refnum<user-event>, error out=w241:errorcluster)
        "tcp data event" <- w235
        n118 = control-ref of="This VI"() -> (w237:refnum<vi>)
        n119 = register-events(w235) -> ()  [unwired: 2 in, 2 out]
        n120 = call "supergui create stop queue.vi"() -> ("STOP Queue out"=w243:refnum<queue>)  [unwired: 11 in]
        n121 = Current VI's Menubar() -> (w236:refnum<k9>)
        n122 = call-by-ref "Start Asynchronous Call"(reference=w247, error in=w246, "STOP Queue in"=w243, "This Application"=w238, 8:"error in (no error)"=w241, "tcp data event"=w235, "Caller menu reference"=w236, "Caller VI ref"=w237) -> (reference out=w230:refnum<vi>, error out=w233:errorcluster)  [unwired: 5 in, 1 out]
        n123 = Bundle By Name(cluster=w240, "SuperGUI.SuperGUI ref"=w230, "SuperGUI.STOP queue"=w243) -> (w239:T17)
        n124 = call <vilib>:"Add State(s) to Queue__jki_lib_state_machine.vi"("State(s) in (\"\")"=w249) -> ("States Out"=w248:string)  [unwired: 14 in]
      }
      frame "UI: Stop SuperGUI" {
        # "Stop Supergui Clone and wait until it exit properly"
        n125 = call <vilib>:"Add State(s) to Queue__jki_lib_state_machine.vi"("State(s) in (\"\")"=w257) -> ("States Out"=w256:string)  [unwired: 14 in]
        n126 = Unbundle By Name(w252) -> ("SuperGUI.SuperGUI ref"=w254:refnum<vi>, "SuperGUI.STOP queue"=w253:refnum<queue>)
        n127 = Release Queue(queue=w253, error in (no error)=w251) -> (error out=w255:errorcluster)  [unwired: 1 in, 2 out]
        n128 = call-by-ref "Wait On Asynchronous Call"(reference=w254, error in=w255) -> ("error out"=w250:errorcluster)  [unwired: 11 in, 2 out]
      }
      frame "UI: Cursor Set" {
        # "Argument"
        # "Set and Unset Cursor Busy.\n(Usage: \"UI: Cursor Set >> Busy|Idle\")"
        n129 = call <vilib>:"Add State(s) to Queue__jki_lib_state_machine.vi"("State(s) in (\"\")"=w263) -> ("States Out"=w262:string)  [unwired: 14 in]
        n130 = case shown="\"Idle\", Default" w258 {
          tunnel: w260 -> [w265 w267]
          tunnel: [w264 w266] -> w259
          frame "Idle", Default {
            n131 = call <vilib>:"Unset Busy.vi"("error in (no error)"=w265) -> ("error out"=w264:errorcluster)  [unwired: 10 in]
          }
          frame "Busy" {
            n132 = call <vilib>:"Set Busy.vi"("error in (no error)"=w267) -> ("error out"=w266:errorcluster)  [unwired: 9 in, 1 out]
          }
        }
      }
      frame "UI: Front Panel State" {
        # "Argument"
        # "Set Front Panel Open or Closed\n(Usage: \"UI: Front Panel State >> Open|Close\")"
        n133 = call <vilib>:"Add State(s) to Queue__jki_lib_state_machine.vi"("State(s) in (\"\")"=w274) -> ("States Out"=w273:string)  [unwired: 14 in]
        n134 = Unbundle By Name(w270) -> ("Core.Current VI Reference"=w269:refnum<vi>)
        n135 = case shown="\"Open\", Default" w268 {
          tunnel: w272 -> [w278 w291]
          tunnel: [w280 w292] -> w271
          tunnel: w269 -> [w279 w289]
          frame "Open", Default {
            n136 = property class="VI"(reference=w279, error in=w278) -> (reference out=w276:refnum<vi>, error out=w277:errorcluster, "Front Panel.Open"=w275:bool)
            n137 = case shown="False" w275 {
              tunnel: [w283 w286] -> w280
              tunnel: w277 -> [w282 w286]
              tunnel: w276 -> [w281 _]
              frame False {
                n138 = invoke class="VI" method="FP.Open"(reference=w281, error in=w282, "Activate"=TRUE, "State"=T16."Standard") -> (error out=w283:errorcluster)  [unwired: 1 in, 4 out]
              }
              frame True {
              }
            }
          }
          frame "Close" {
            n139 = property class="VI"(reference=w289, error in=w291) -> (reference out=w288:refnum<vi>, error out=w290:errorcluster, "Front Panel.Open"=w287:bool)
            n140 = case shown="True" w287 {
              tunnel: [w293 w296] -> w292
              tunnel: w290 -> [w293 w295]
              tunnel: w288 -> [_ w294]
              frame False {
              }
              frame True {
                n141 = invoke class="VI" method="FP.Close"(reference=w294, error in=w295) -> (error out=w296:errorcluster)  [unwired: 1 in, 2 out]
              }
            }
          }
        }
      }
      frame "---------- Macro ----------" {
        # "Do not put any code in this frame.\n(It is a separator no-op. You can make a copy of this frame to create a new Macro frame)"
        n142 = call <vilib>:"Add State(s) to Queue__jki_lib_state_machine.vi"("State(s) in (\"\")"=w300) -> ("States Out"=w299:string)  [unwired: 14 in]
      }
      frame "Macro: Initialize" {
        # "Initialization Macro\n(This is called once, when the VI starts)"
        n143 = call <vilib>:"Add State(s) to Queue__jki_lib_state_machine.vi"("State(s) in Front (\"\")"="Data: Initialize\nInitialize Core Data\nUI: Initialize\nUI: Get Device Name\nUI: Start SuperGUI\nUI: Front Panel State >> Open", "State(s) in (\"\")"=w305) -> ("States Out"=w304:string)  [unwired: 13 in]
      }
      frame "Macro: Exit" {
        # "Exit Macro\n(This is called once, when the VI exits)"
        n144 = Unbundle By Name(w313) -> ("Core.Close Panel on Exit?"=w312:bool)
        n145 = Select(t="UI: Front Panel State >> Close", s=w312, f="") -> (s? t:f=w309:string)
        n146 = call <vilib>:"Add State(s) to Queue__jki_lib_state_machine.vi"("State(s) in Front (\"\")"="UI: Stop SuperGUI" ("State(s) in Front (\"\")"), "State(s) in (\"\")"=w309, "State(s) at Back (\"\")"="Data: Cleanup\nExit") -> ("States Out"=w307:string)  [unwired: 12 in]
        n147 = call <vilib>:"Add State(s) to Queue__jki_lib_state_machine.vi"("State(s) in Front (\"\")"=w307, "State(s) in (\"\")"=w316) -> ("States Out"=w315:string)  [unwired: 13 in]
      }
      frame "---------- New Category ----------" {
        # "Template Separator\n(You can make a copy of, or modify, this frame)"
        n148 = call <vilib>:"Add State(s) to Queue__jki_lib_state_machine.vi"("State(s) in (\"\")"=w320) -> ("States Out"=w319:string)  [unwired: 14 in]
      }
      frame "New Category: 1" {
        # "Your code here.\n(You can make a copy of, or modify, this frame)"
        n149 = call <vilib>:"Add State(s) to Queue__jki_lib_state_machine.vi"("State(s) in (\"\")"=w324) -> ("States Out"=w323:string)  [unwired: 14 in]
      }
      frame "New Category: 2" {
        # "Your code here.\n(You can make a copy of, or modify, this frame)"
        n150 = call <vilib>:"Add State(s) to Queue__jki_lib_state_machine.vi"("State(s) in (\"\")"=w328) -> ("States Out"=w327:string)  [unwired: 14 in]
      }
    }
  }
